vi "Euler_ang2quat RAD(SubVI).vi"(11 "Euler Angles [rad]":cluster{"phi":dbl, "theta":dbl, "psi":dbl}) -> (3 "Quaternions":dbl[](array[numeric]))   [LabVIEW 2017]
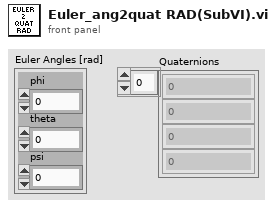
[diagram p1: front panel]
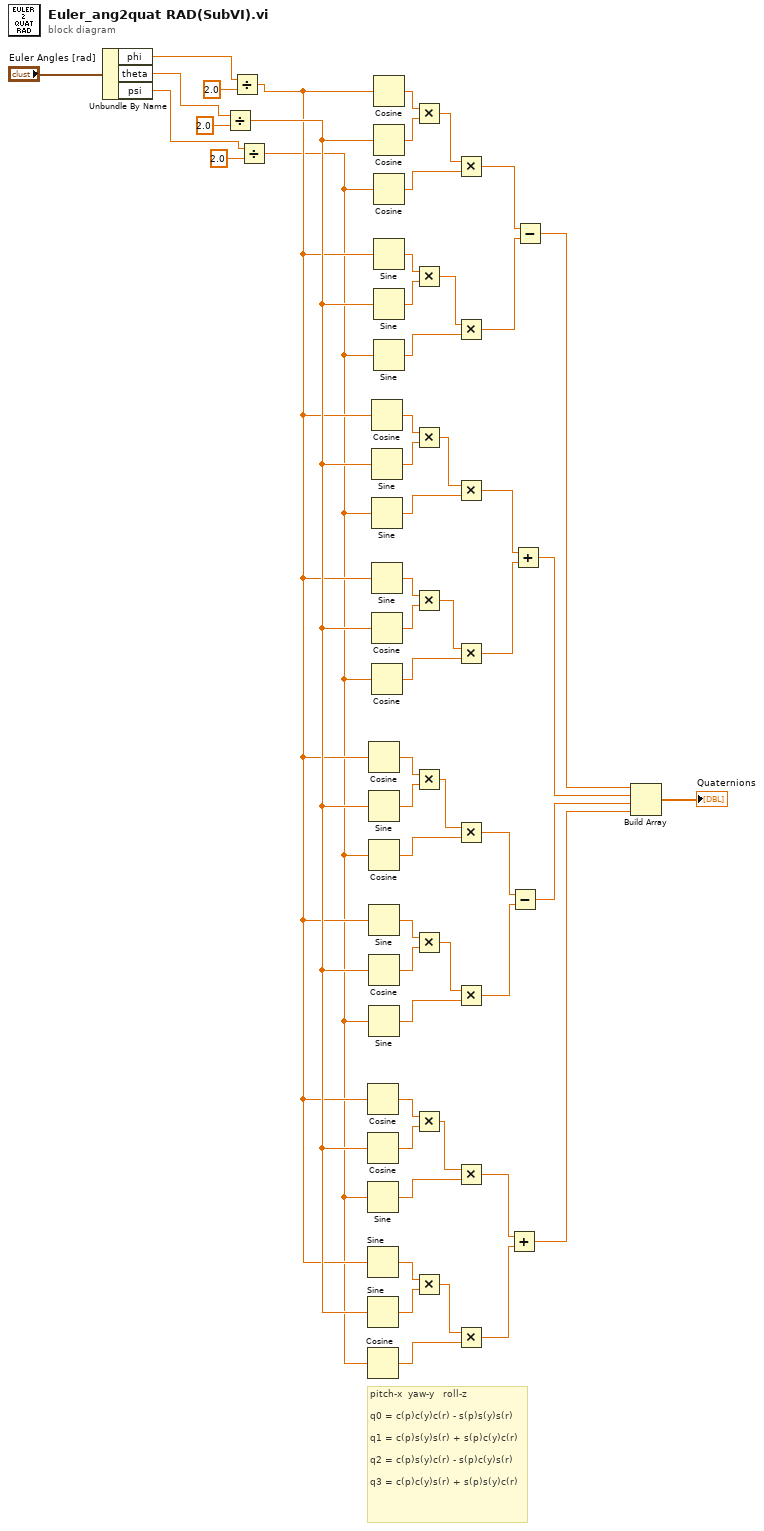
[diagram p0: block diagram]
diagram:
  # "pitch-x  yaw-y   roll-z\n\nq0 = c(p)c(y)c(r) - s(p)s(y)s(r)\n\nq1 = c(p)s(y)s(r) + s(p)c(y)c(r)\n\nq2 = c(p)s(y)c(r) - s(p)c(y)s(r)\n\nq3 = c(p)c(y)s(r) + s(p)s(y)c(r)"
  n1 = Unbundle By Name("Euler Angles [rad]") -> ("phi"=w3:dbl, "theta"=w2:dbl, "psi"=w1:dbl)
  n2 = Divide(x=w2, y=2.0) -> (x/y=w55:dbl)
  n3 = Divide(x=w3, y=2.0) -> (x/y=w53:dbl)
  n4 = Divide(x=w1, y=2.0) -> (x/y=w5:dbl)
  n5 = Cosine(x=w53) -> (cos(x)=w46:dbl)
  n6 = Cosine(x=w55) -> (cos(x)=w45:dbl)
  n7 = Sine(x=w5) -> (sin(x)=w43:dbl)
  n8 = Sine(x=w53) -> (sin(x)=w41:dbl)
  n9 = Sine(x=w55) -> (sin(x)=w40:dbl)
  n10 = Cosine(x=w5) -> (cos(x)=w39:dbl)
  n11 = Cosine(x=w53) -> (cos(x)=w27:dbl)
  n12 = Sine(x=w55) -> (sin(x)=w28:dbl)
  n13 = Cosine(x=w5) -> (cos(x)=w30:dbl)
  n14 = Sine(x=w53) -> (sin(x)=w32:dbl)
  n15 = Cosine(x=w55) -> (cos(x)=w33:dbl)
  n16 = Sine(x=w5) -> (sin(x)=w34:dbl)
  n17 = Cosine(x=w53) -> (cos(x)=w26:dbl)
  n18 = Sine(x=w55) -> (sin(x)=w25:dbl)
  n19 = Sine(x=w5) -> (sin(x)=w23:dbl)
  n20 = Sine(x=w53) -> (sin(x)=w21:dbl)
  n21 = Cosine(x=w55) -> (cos(x)=w20:dbl)
  n22 = Cosine(x=w5) -> (cos(x)=w19:dbl)
  n23 = Cosine(x=w53) -> (cos(x)=w7:dbl)
  n24 = Cosine(x=w55) -> (cos(x)=w8:dbl)
  n25 = Cosine(x=w5) -> (cos(x)=w10:dbl)
  n26 = Sine(x=w53) -> (sin(x)=w12:dbl)
  n27 = Sine(x=w55) -> (sin(x)=w13:dbl)
  n28 = Sine(x=w5) -> (sin(x)=w14:dbl)
  n29 = Multiply(x=w7, y=w8) -> (x*y=w9:dbl)
  n30 = Multiply(x=w12, y=w13) -> (x*y=w11:dbl)
  n31 = Multiply(x=w26, y=w25) -> (x*y=w24:dbl)
  n32 = Multiply(x=w21, y=w20) -> (x*y=w22:dbl)
  n33 = Multiply(x=w27, y=w28) -> (x*y=w29:dbl)
  n34 = Multiply(x=w32, y=w33) -> (x*y=w31:dbl)
  n35 = Multiply(x=w46, y=w45) -> (x*y=w44:dbl)
  n36 = Multiply(x=w41, y=w40) -> (x*y=w42:dbl)
  n37 = Multiply(x=w9, y=w10) -> (x*y=w15:dbl)
  n38 = Multiply(x=w11, y=w14) -> (x*y=w16:dbl)
  n39 = Multiply(x=w24, y=w23) -> (x*y=w18:dbl)
  n40 = Multiply(x=w22, y=w19) -> (x*y=w17:dbl)
  n41 = Multiply(x=w29, y=w30) -> (x*y=w35:dbl)
  n42 = Multiply(x=w31, y=w34) -> (x*y=w36:dbl)
  n43 = Multiply(x=w44, y=w43) -> (x*y=w38:dbl)
  n44 = Multiply(x=w42, y=w39) -> (x*y=w37:dbl)
  n45 = Add(x=w38, y=w37) -> (x+y=w50:dbl)
  n46 = Subtract(x=w35, y=w36) -> (x-y=w49:dbl)
  n47 = Add(x=w18, y=w17) -> (x+y=w48:dbl)
  n48 = Subtract(x=w15, y=w16) -> (x-y=w47:dbl)
  n49 = Build Array(w47, w48, w49, w50) -> (→"Quaternions":dbl[])
